vi "CPP-7021Polar.vi"(0 "Plot Array":cluster{dbl[], dbl[]}[](array[cluster])=[{[500.0, 500.0, 953.54, 215.0, 270.0, 320.0, 445.0, 525.0, 600.0, 675.0, 750.0, 825.0, 900.0, 960.0, 1010.0, 1060.0], [4.614524, 4.54365, 5.818368, 0.1374656, 0.6662545, 1.465458, 3.619824, 4.848976, 5.887329, 5.940571, 6.152151, 5.717487, 5.600293, 5.40069, 5.154843, 5.121789]}, {[100.0, 150.0, 215.0, 270.0, 320.0, 445.0, 525.0, 600.0, 675.0, 750.0, 825.0, 900.0, 960.0, 1010.0, 1060.0], [0.002314715, -0.00693192, 0.120417, 0.6880509, 1.519176, 3.513709, 5.065183, 6.116033, 6.096773, 5.938465, 5.593788, 5.5597, 5.387002, 5.304077, 4.887903]}] {"?" format="%.2f"; "?" format="%.2f"}, 1 "Job Directory":path=path "/G4_2_HD/Users/paulhayden/Documents/Projects/Westlakes_resolution") -> (2 "Saved Automatically?":bool, 3 "gnuplotScript":string="set term epslatex\nset output \"Plot.eps\"\nset xlabel '$Distance~(m)$'\nset ylabel '$DF~(s/m^3)\\times10^6$'\nset samples 1000\nset pointsize 1.00\nset title '$B38~Centreline~Glc$' 0, 0\nset size 0.75,0.9\n\n#set key 450, -2.5833\n unset key\nset label 1 '~~~~~~~~~~~Angle~(deg)~=~0' at -100, -2.58\nset label 2 '~~~~~~~~~~~Height~(m)~=~5' at -100, -3.27\n set xrange [0 : 500] \n# set autoscale x \n set yrange [0.10000 : 7]\n# set autoscale y \n\nplot \"B38_Centreline_Glc.dat\" index 0 using 1:2 axes x1y1 title '$File=B38R~DDD.xls$' with points 1 1, \\\n\"B38_Centreline_Glc.dat\" index 1 using 1:2 axes x1y1 title '$File=B38R~DDD~1.xls$' with points 1 3", 4 "Plot data file":path)   [LabVIEW 2015]
uses:
  Results_plotter_Global.vi
panel:
  in  "Tab Control":enum32{"GoodStuff", "OtherStuff"}(tab)
  in  "Margins":dbl=0.6 min=0.1 max=2.0 step=0.1
  out "No of Series":i32=2
  in  "PropertyArray":T1(array[cluster])=[{"Style"="lines", "Color"=16711680, "PointType"=2, "PointSize"=0.6}, {"Style"="points", "Color"=16860, "PointType"=6, "PointSize"=0.6}, {"Style"="points", "Color"=1985280, "PointType"=5, "PointSize"=0.6}, {"Style"="lines", "Color"=0, "PointType"=5, "PointSize"=0.6}] caption="Style                      Colour    PointType       PointSize" {"PointSize" min=0 step=0.1}
  in  "Rows":u8=4 min=1
  in  "Cols":u8=6 min=1
  out "nGraphs":i32
  in  "rmax":dbl=1.1 step=0.1
  in  "rtics":dbl=0.2 step=0.1
  in  "ManualTitles":string[](array[string])=["", "", "", "", "", "", "", "", "", "", "", "", "", "", "", ""]
  in  "Titles":bool=TRUE
  in  "ScaleFactor":dbl
  in  "ScaleAdjust":dbl=0.1 min=0.1 max=2.0 step=0.1
  in  "Legend?":bool
  in  "AngleTics":dbl=30.0 step=0.1
  in  "r Axis?":bool
  in  "Plot Title Pre Block":string
  in  "Plot Title":u16(ring) items=["Title String Only", "Number of Measurements", "TT:used:", "Fence::", "Comments::", "Azimuth::", "ExtraNotes::", "X::", "Y::", "Z_{model}::", "U/Uref::", "U/U(167)::", "(U/Uref)-1::", "V/Uref::", "W/Uref::", "Vmag/Uref::", "Uref::", "U::", "V::", "W::", "Vmag::", "TI:U:%", "TI:V:%", "TI:W:%", "TI:Vmag:%", "Upk/Upk(167)::", "Vmagpk/Uref::", "U_SD::", "V_SD::", "W_SD::", "Vmag_SD::", "Tunnel:X:", "Tunnel:Y:", "5HP:Mode:", "5HP:ReturnType:", "GoodFraction::", "DownstreamEars::", "Ramps::", "Reference:Temperature:Used for Corrections", "Atmos:Pressure:Used for Corrections", "Seconds:since:1st Jan", "Time:Measurement:Commenced", "Multi Run:Start Time:", "Date:of:Measurement", "Run:Messages:", "Current:Data:Filename", "Original:Results:Filename", "Raw:Data:Filename", "P1:mm:", "PostProcessBatch::", "Upk(z=167,Base,AllPts,AllAzs)/Uref::", "U(z=167,Base,AllPts,AllAzs)/Uref::", "Horizontal~Velocity/U_{ref}::", "Z_{fs}:(m):"]
  in  "Plot Title Post Block":string
  out "Array":string[](array[string])
  in  "OpenLogfile?":bool
  in  "Filename Max length":i32=255
  in  "Show Script Editor?":bool
  out "Path":path
  out "Final Title":string="B38 Centreline Glc"
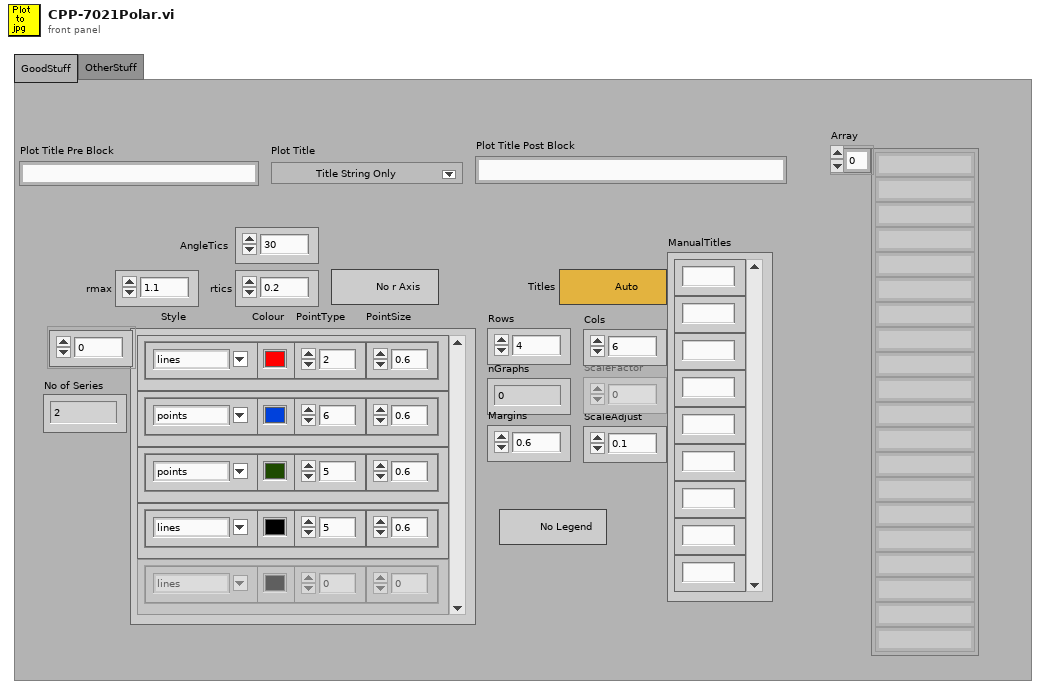
[diagram p1: front panel]
types:
  T1 = cluster{"Style":string, "Color":u32, "PointType":i32, "PointSize":sgl}[]
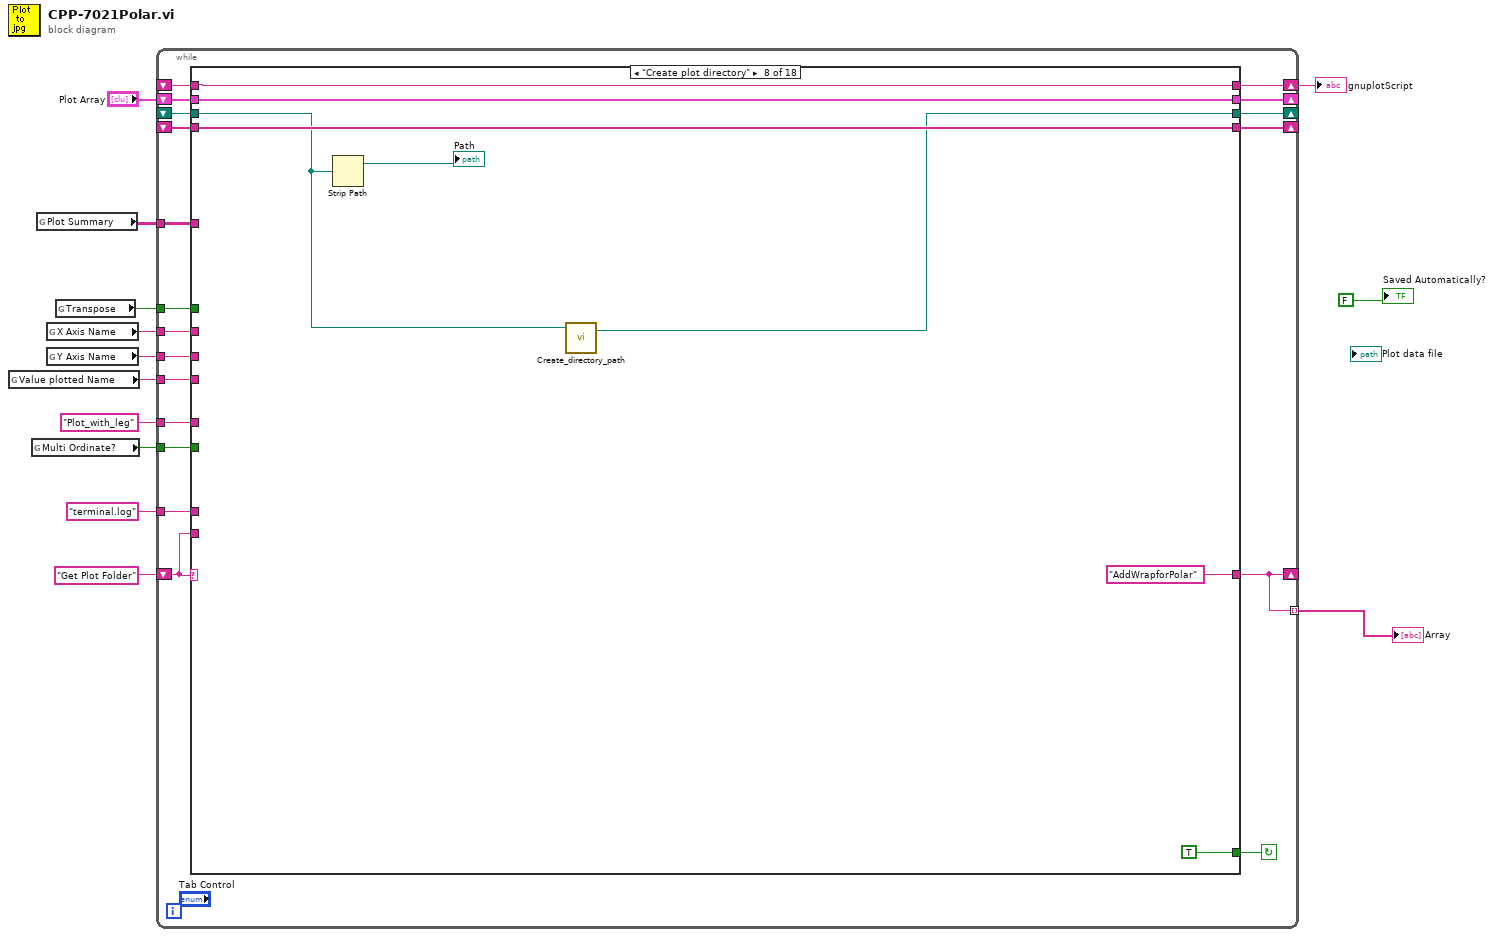
[diagram p0: block diagram]
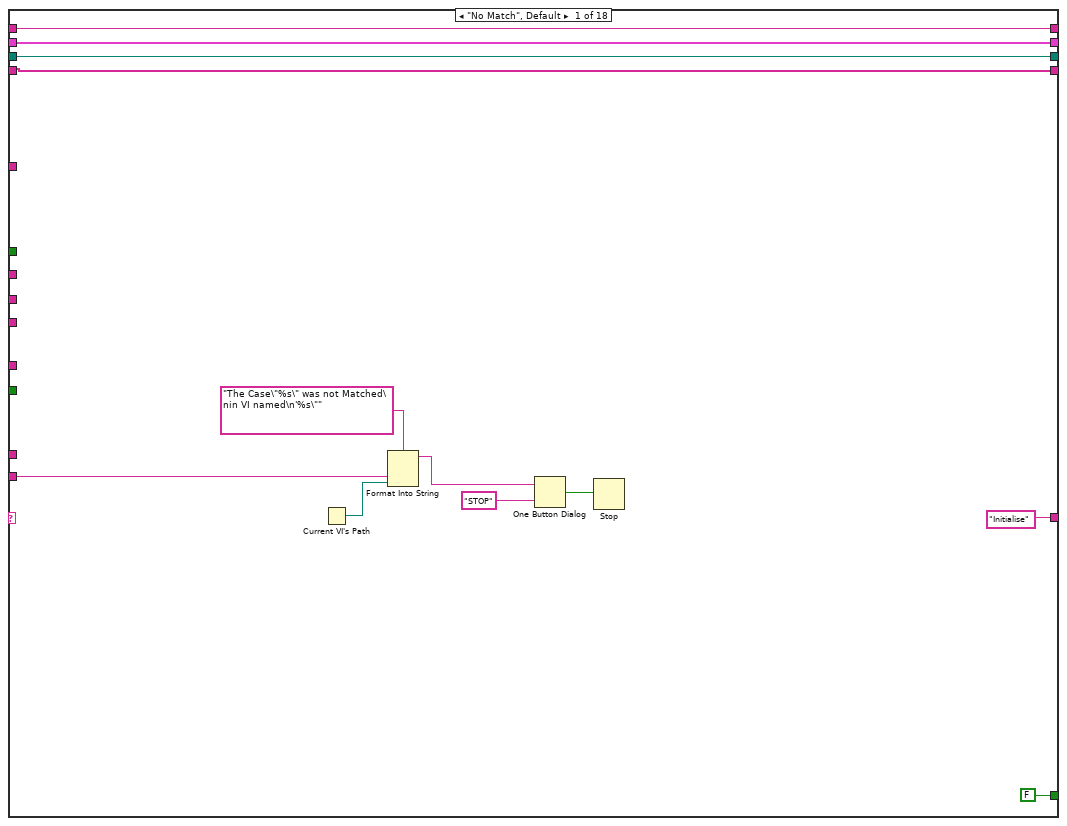
[diagram p2: hidden frame]
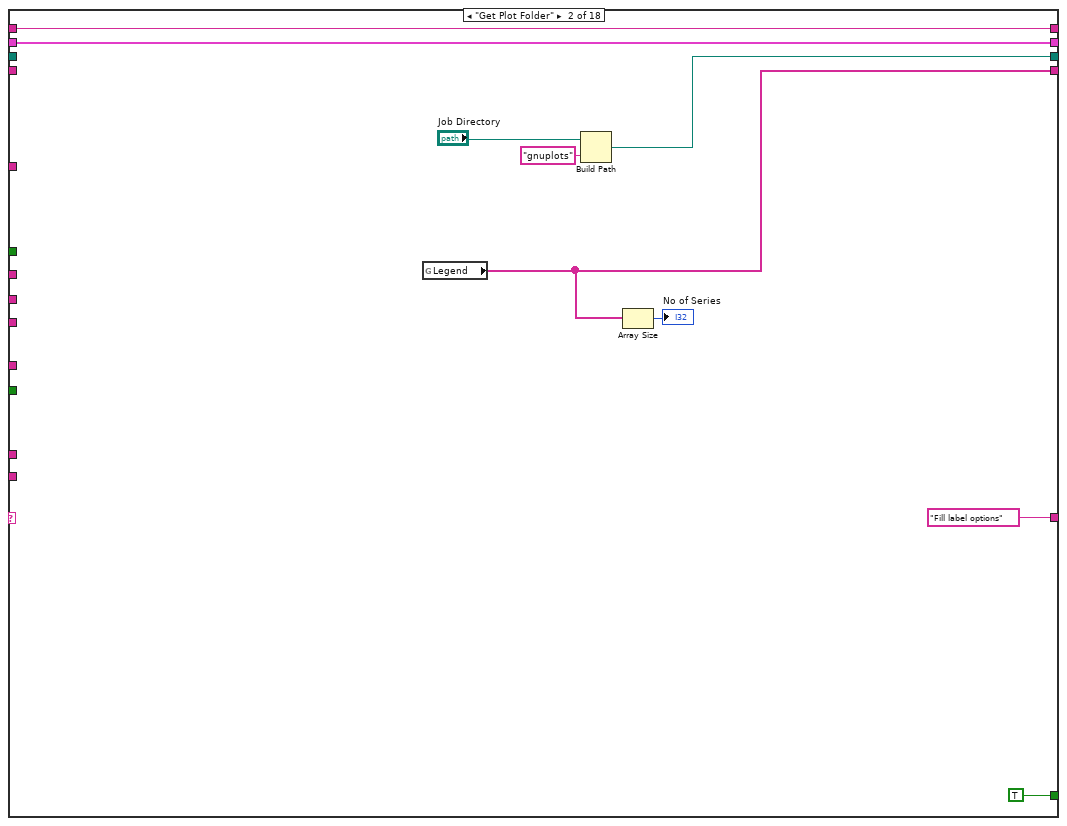
[diagram p3: hidden frame]
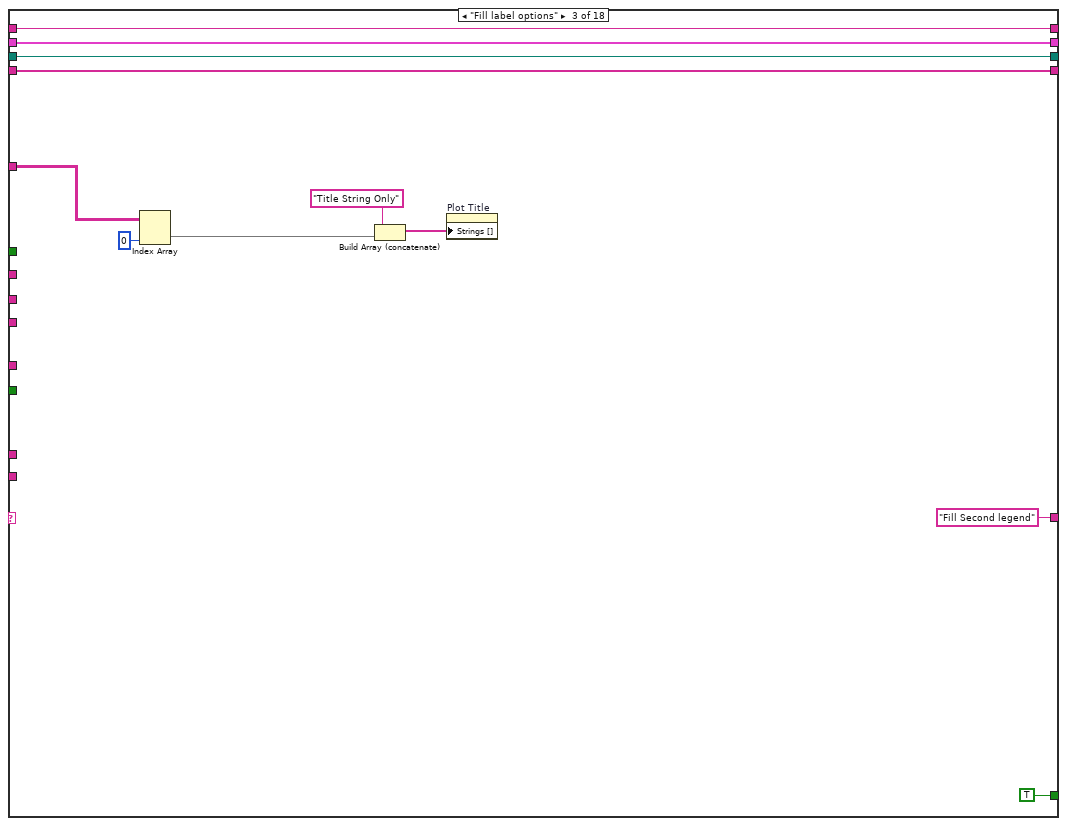
[diagram p4: hidden frame]
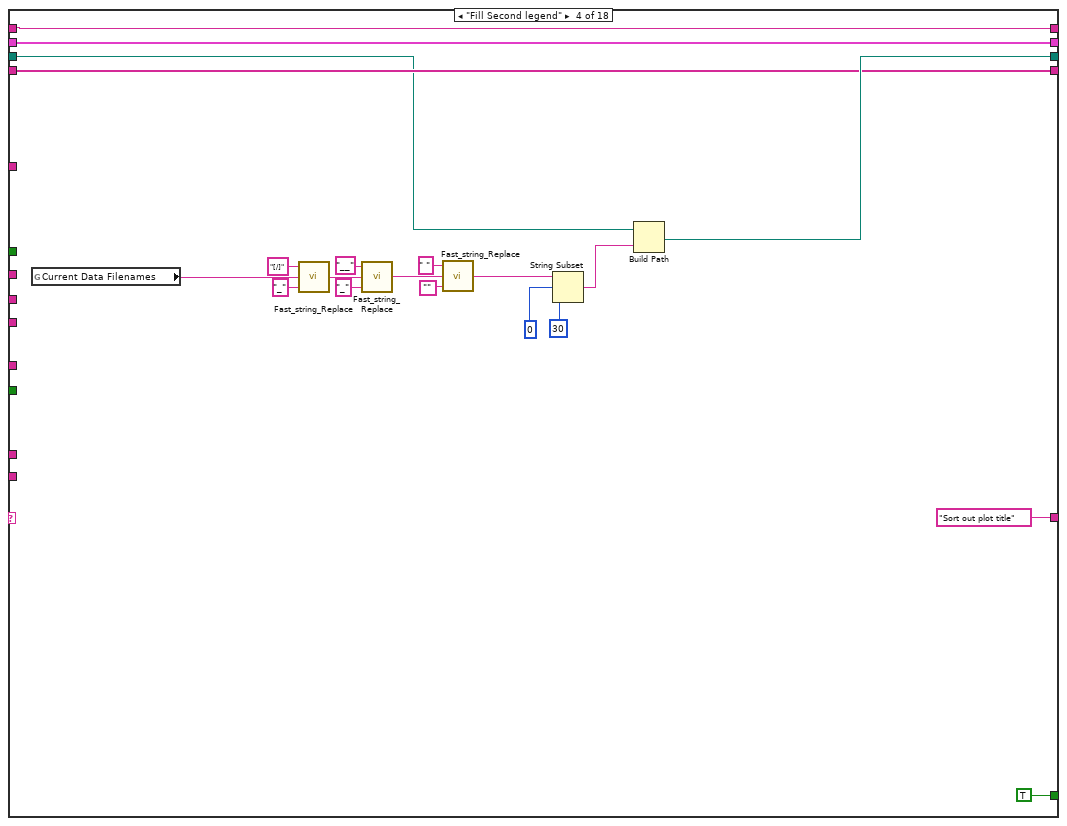
[diagram p5: hidden frame]
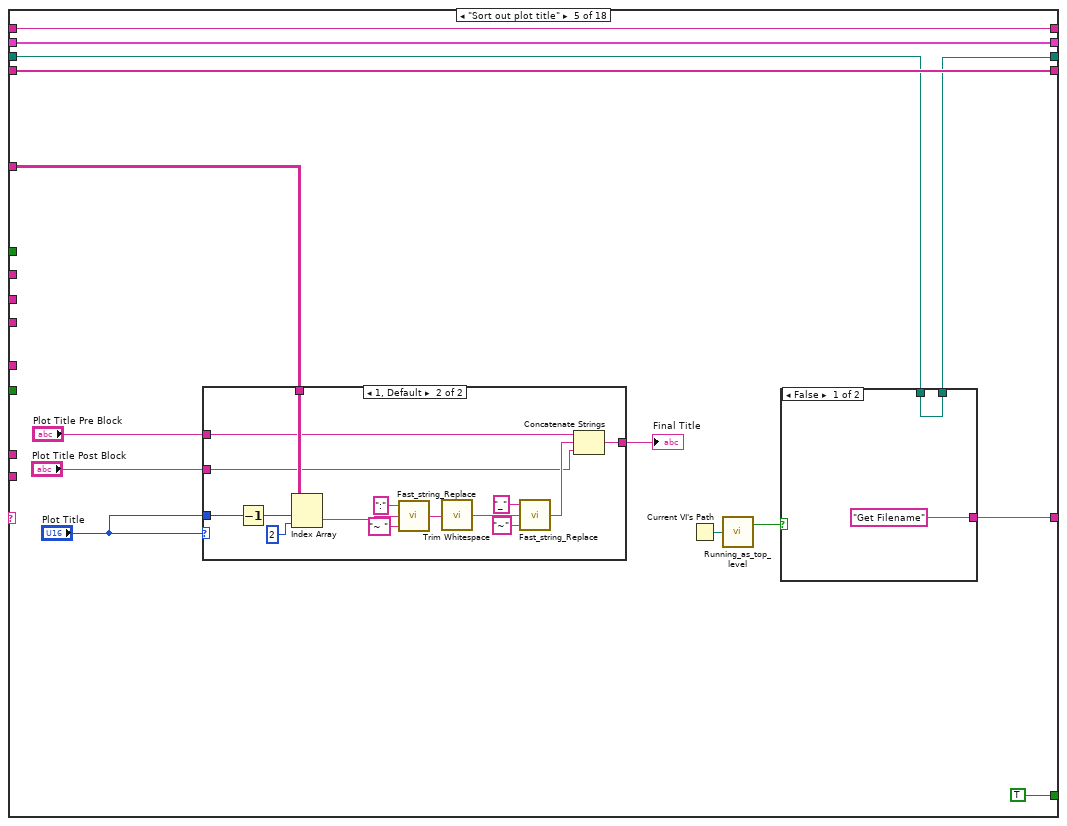
[diagram p6: hidden frame]
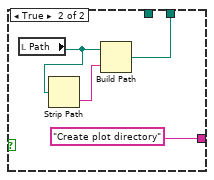
[diagram p7: hidden frame]
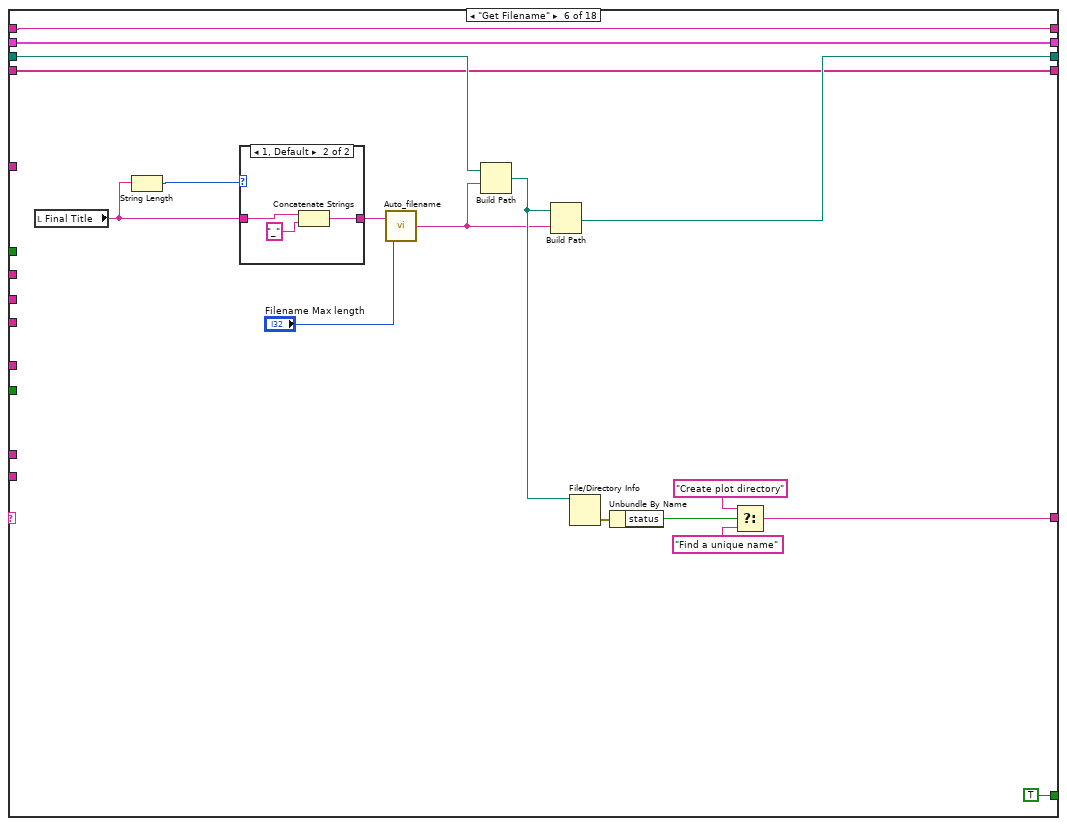
[diagram p9: hidden frame]
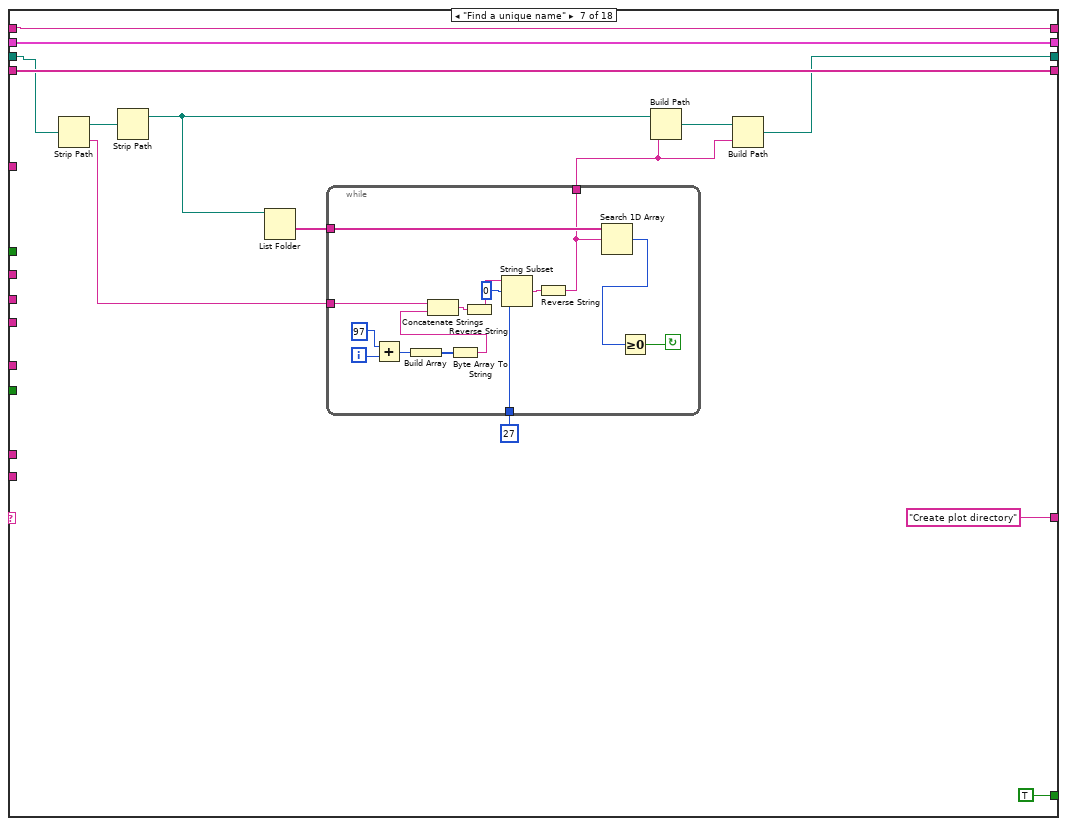
[diagram p11: hidden frame]
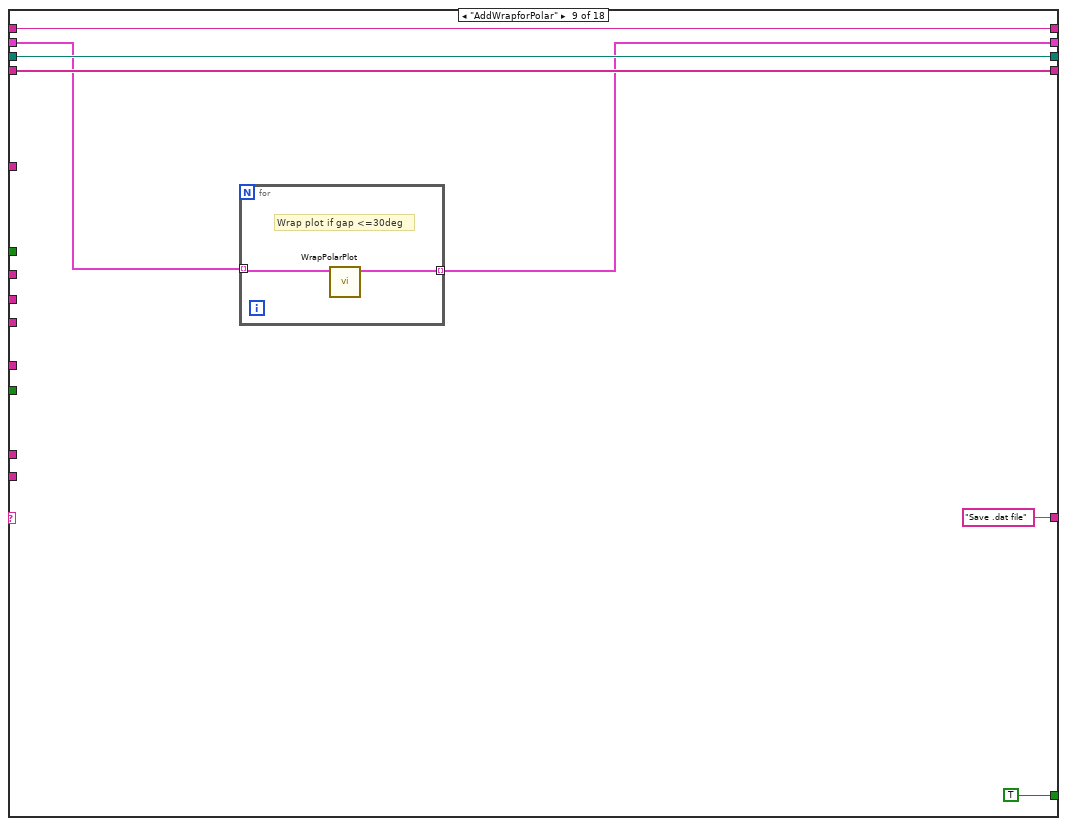
[diagram p12: hidden frame]
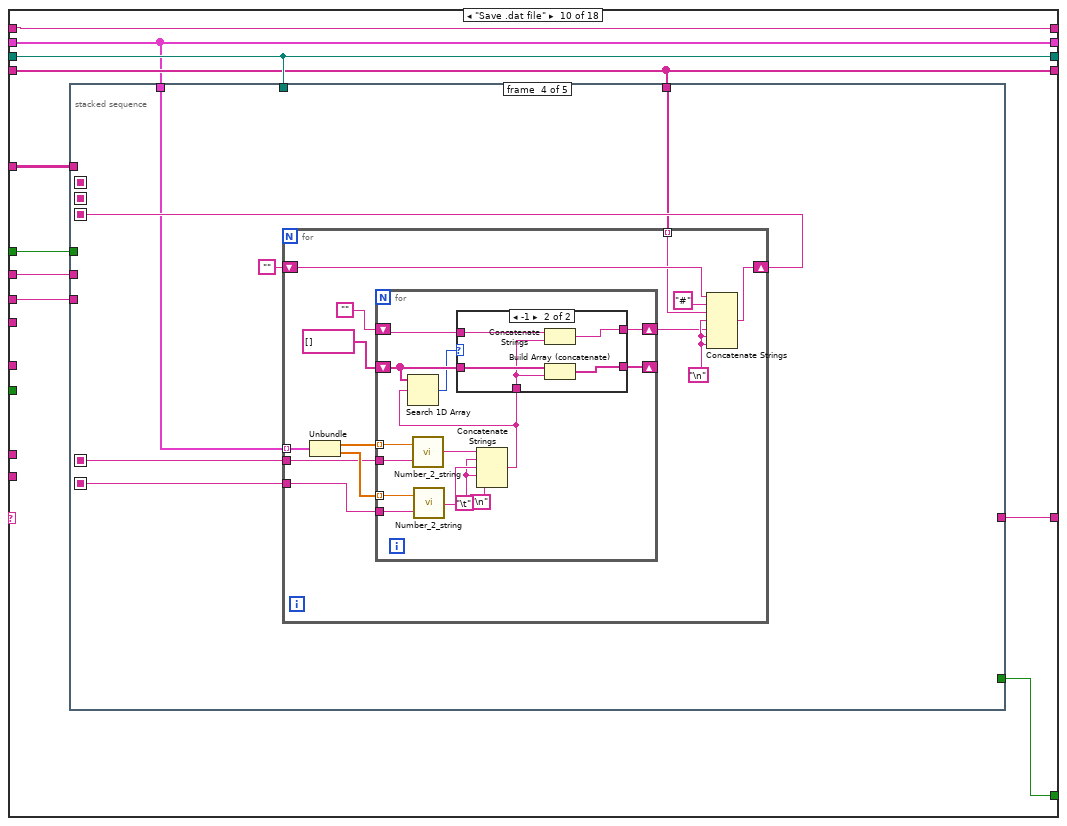
[diagram p13: hidden frame]
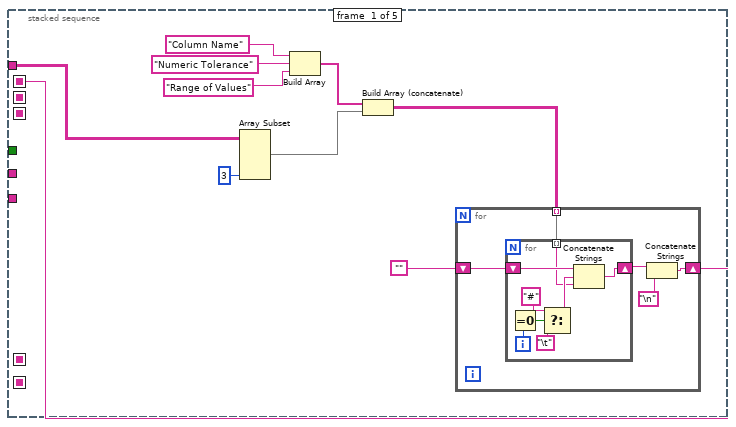
[diagram p14: hidden frame]
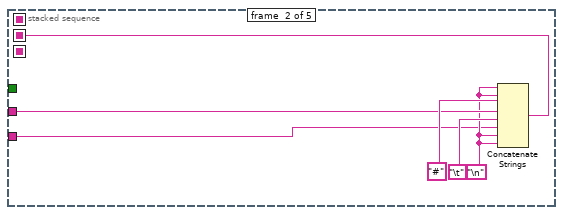
[diagram p15: hidden frame]
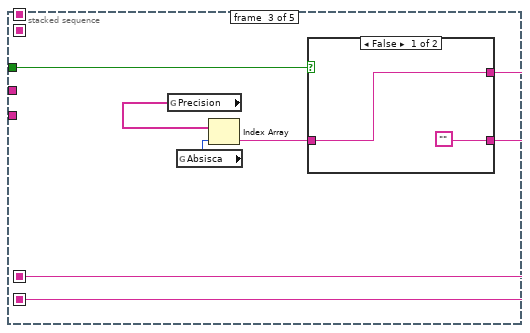
[diagram p16: hidden frame]
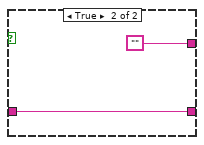
[diagram p17: hidden frame]
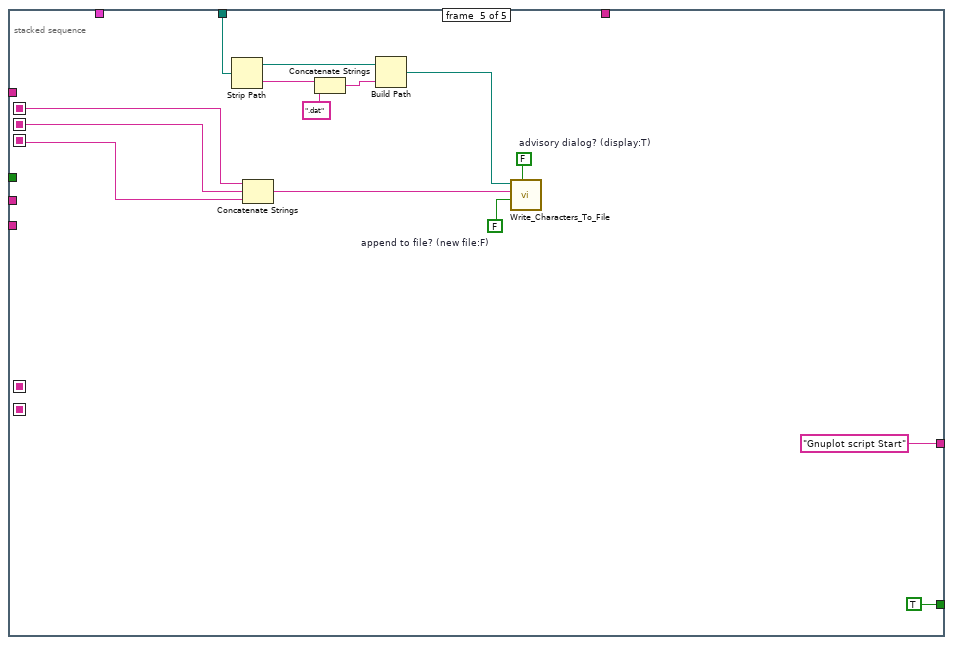
[diagram p19: hidden frame]
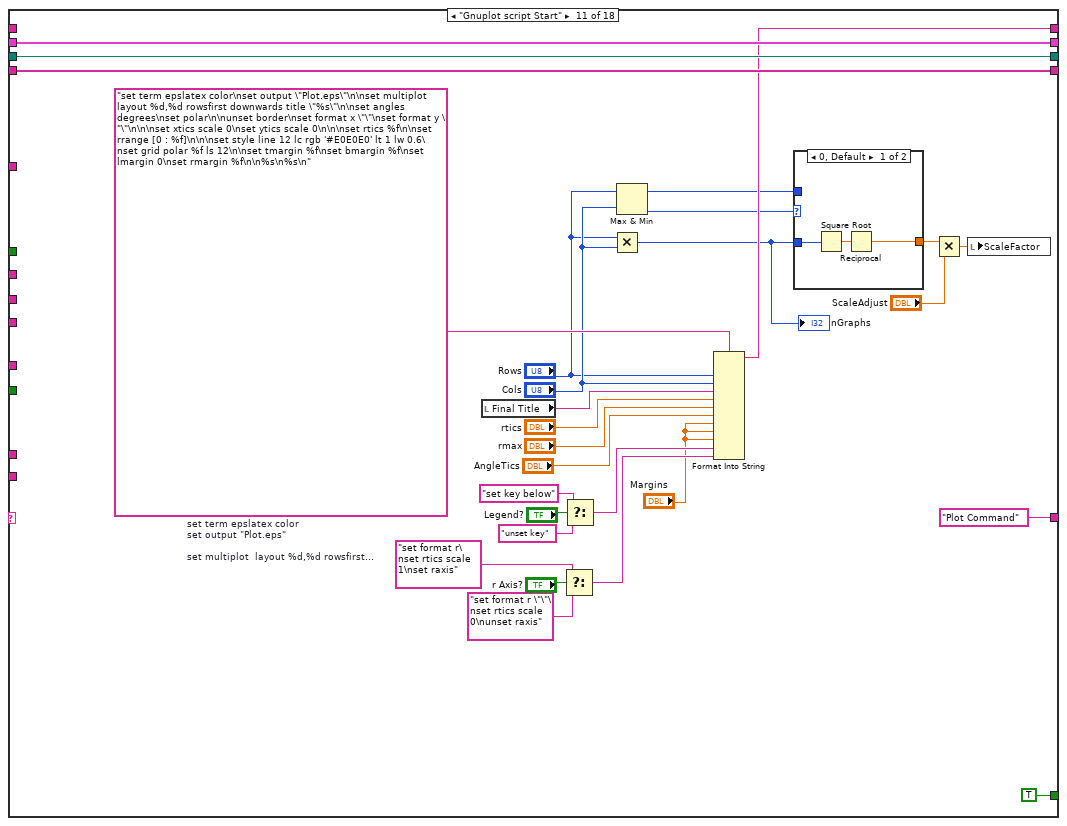
[diagram p20: hidden frame]
diagram:
  n1 = global read "Results_plotter_Global.vi" "Value plotted Name"() -> (w9:string)
  n2 = global read "Results_plotter_Global.vi" "Multi Ordinate?"() -> (w2:bool)
  n3 = global read "Results_plotter_Global.vi" "Plot Summary"() -> (w12:string[][])
  n4 = global read "Results_plotter_Global.vi" "X Axis Name"() -> (w11:string)
  n5 = global read "Results_plotter_Global.vi" "Y Axis Name"() -> (w10:string)
  n6 = global read "Results_plotter_Global.vi" "Transpose"() -> (w3:bool)
  n7 = while {
    shift-left: "Get Plot Folder" -> [w31]
    shift-right: [w14] -> _
    tunnel: w12 -> [w30]
    shift-right: [w29] -> _
    shift-left: _ -> [w28]
    tunnel: w11 -> [w27]
    tunnel: w10 -> [w26]
    tunnel: w9 -> [w25]
    shift-right: [w23] -> _
    shift-left: "Plot Array" -> [w24]
    shift-right: [w21] -> w8
    shift-left: _ -> [w22]
    tunnel: "Plot_with_leg" ("name or relative path") -> [w20]
    shift-right: [w19] -> _
    shift-left: _ -> [w18]
    tunnel: "terminal.log" -> [w17]
    tunnel: w3 -> [w16]
    tunnel: w2 -> [w15]
    tunnel: [w14] -> w1 mode=indexing
    stop <- w32 continue-if-true
    n8 = case shown="\"Create plot directory\"" w31 {
      tunnel: [FALSE TRUE TRUE ("Top Level") TRUE ("Top Level") TRUE ("Top Level") TRUE ("Top Level") TRUE ("Top Level") TRUE TRUE ("Top Level") w195 TRUE ("Top Level") TRUE ("Top Level") TRUE ("Top Level") TRUE ("Top Level") TRUE ("Top Level") FALSE ("Top Level") FALSE ("Top Level") FALSE ("Top Level")] -> w32
      tunnel: ["Initialise" "Fill label options" "Fill Second legend" "Sort out plot title" w86 w135 "Create plot directory" "AddWrapforPolar" "Save .dat file" w194 "Plot Command" "Write gnuplot file" ("t") "Execute shell script" ("t") "Has pdf been generated?" ("t") w429 "End" "End" ("t") "End" ("t")] -> w14
      tunnel: w31 -> [w39 _ _ _ _ _ _ _ _ _ _ _ _ _ _ _ _ _]
      tunnel: w30 -> [_ _ w64 _ w93 _ _ _ _ w193 _ _ _ _ _ _ _ _]
      tunnel: [w36 w50 w58 w84 w88 w136 w142 w175 w184 w196 w317 w341 w411 w419 w433 w438 w448 w454] -> w29
      tunnel: w28 -> [w36 _ w58 w80 w87 w132 w149 w174 w184 w196 w317 w341 w411 w419 w433 w438 w448 w454]
      tunnel: w27 -> [_ _ _ _ _ _ _ _ _ w192 _ _ _ _ _ _ _ _]
      tunnel: w26 -> [_ _ _ _ _ _ _ _ _ w191 _ _ _ _ _ _ _ _]
      tunnel: w25 -> [_ _ _ _ _ _ _ _ _ _ _ _ _ _ _ _ _ _]
      tunnel: w24 -> [w35 w46 w59 w83 w98 w134 w152 w178 w180 w188 w318 w342 w417 w424 w436 w443 w453 w459]
      tunnel: [w35 w46 w59 w83 w98 w134 w152 w178 w179 w188 w318 w342 w417 w424 w436 w443 w453 w459] -> w23
      tunnel: w22 -> [w34 w49 w60 w82 w94 w133 w151 w177 w185 w197 _ w339 w407 w422 w434 w441 w451 w457]
      tunnel: [w34 w49 w60 w82 w94 w133 w151 w177 w185 w197 w312 w338 w407 w422 w434 w441 w451 w457] -> w21
      tunnel: w20 -> [_ _ _ _ _ _ _ _ _ _ _ _ _ _ _ _ _ _]
      tunnel: [w33 w45 w57 w81 w97 w131 w150 w176 w183 w190 w316 w340 w412 w423 w435 w442 w452 w458] -> w19
      tunnel: w18 -> [w33 _ w57 w81 w97 w131 w150 w176 w183 w190 w316 w340 w412 w423 w435 w442 w452 w458]
      tunnel: w17 -> [_ _ _ _ _ _ _ _ _ _ _ _ _ w418 _ _ w446 _]
      tunnel: w16 -> [_ _ _ _ _ _ _ _ _ w189 _ _ _ _ _ _ _ _]
      tunnel: w15 -> [_ _ _ _ _ _ _ _ _ _ _ _ _ _ _ _ _ _]
      frame "No Match", Default {
        n9 = Current VI's Path() -> (path=w38:path)
        n10 = Format Into String(format string="The Case\"%s\" was not Matched\nin VI named\n'%s\"" ("Format String"), w39, w38) -> (resulting string=w42:string)  [unwired: 2 in, 1 out]
        n11 = One Button Dialog(message=w42, button name ("OK")="STOP") -> (true=w40:bool)
        n12 = Stop(stop? (T)=w40) -> ()
      }
      frame "Get Plot Folder" {
        n13 = global read "Results_plotter_Global.vi" "Legend"() -> (w45:string[])
        n14 = Build Path(base path="Job Directory", name or relative path="gnuplots") -> (appended path=w50:path)
        n15 = Array Size(array=w45) -> (size(s)=→"No of Series":i32)
      }
      frame "Fill label options" {
        n16 = Index Array(array=w64, index (col)=0 ("disabled index (col)")) -> (element=w55:string[])  [unwired: 1 in]
        n17 = Build Array (concatenate)("Title String Only", w55) -> (w54:string[])
        n18 = property on="Plot Title" class="Ring (strict)"("Strings []"=w54) -> ()  [unwired: 2 in, 2 out]
      }
      frame "Fill Second legend" {
        n19 = global read "Results_plotter_Global.vi" "Current Data Filenames"() -> (w69:string)
        n20 = call "Fast_string_Replace.vi"("Replace match with:"="_", "Input String"=w69, "regular expression"="[/]") -> ("Output String"=w73:string)  [unwired: 2 out]
        n21 = call "Fast_string_Replace.vi"("Replace match with:"="_", "Input String"=w73, "regular expression"="__") -> ("Output String"=w70:string)  [unwired: 2 out]
        n22 = call "Fast_string_Replace.vi"("Replace match with:"="", "Input String"=w70, "regular expression"=" ") -> ("Output String"=w68:string)  [unwired: 2 out]
        n23 = String Subset(string=w68, offset (0)=0, length (rest)=30 ("length (rest)")) -> (substring=w67:string)
        n24 = Build Path(base path=w80, name or relative path=w67) -> (appended path=w84:path)
      }
      frame "Sort out plot title" {
        n25 = case shown="1, Default" "Plot Title" {
          tunnel: [w105 w110] -> w92
          tunnel: "Plot Title Pre Block" -> [w105 w109]
          tunnel: w93 -> [_ w113]
          tunnel: "Plot Title" -> [_ w112]
          tunnel: "Plot Title Post Block" -> [_ w106]
          frame 0 {
          }
          frame 1, Default {
            n26 = Decrement(x=w112) -> (x-1=w111:u16)
            n27 = Index Array(array=w113, index (row)=w111, index (col)=u16 2 ("y")) -> (element=w116:string)
            n28 = call "Fast_string_Replace.vi"("Replace match with:"="~ ", "Input String"=w116, "regular expression"=":") -> ("Output String"=w115:string)  [unwired: 2 out]
            n29 = call <vilib>:"Trim Whitespace.vi"("string"=w115) -> ("trimmed string"=w114:string)  [unwired: 1 in]
            n30 = call "Fast_string_Replace.vi"("Replace match with:"="~", "Input String"=w114, "regular expression"="_") -> ("Output String"=w108:string)  [unwired: 2 out]
            n31 = Concatenate Strings(w109, w108, w106) -> (w110:string)
          }
        }
        "Final Title" <- w92
        n32 = Current VI's Path() -> (path=w91:path)
        n33 = call "Running_as_top_level.vi"("Vi path name"=w91) -> ("Top Level"=w89:bool)  [unwired: 1 out]
        n34 = case shown="False" w89 {
          tunnel: [w100 w103] -> w88
          tunnel: w87 -> [w100 _]
          tunnel: ["Get Filename" ("t") "Create plot directory"] -> w86
          frame False {
          }
          frame True {
            n35 = local read "Path"() -> (w102:path)
            n36 = Strip Path(path=w102) -> (name=w101:string)  [unwired: 1 out]
            n37 = Build Path(base path=w102, name or relative path=w101) -> (appended path=w103:path)
          }
        }
      }
      frame "Get Filename" {
        n38 = local read "Final Title"() -> (w121:string)
        n39 = String Length(string=w121) -> (length=w123:i32)
        n40 = case shown="1, Default" w123 {
          tunnel: [w138 w139] -> w122
          tunnel: w121 -> [w138 w141]
          frame 0 {
          }
          frame 1, Default {
            n41 = Concatenate Strings(w141, "_") -> (w139:string)
          }
        }
        n42 = call "Auto_filename.vi"("Filename Max length"="Filename Max length", "Prefix"=w122) -> ("Filename"=w125:string)
        n43 = Build Path(base path=w132, name or relative path=w125) -> (appended path=w129:path)
        n44 = Build Path(base path=w129, name or relative path=w125) -> (appended path=w136:path)
        n45 = File/Directory Info(path=w129) -> (error out=w130:errorcluster)  [unwired: 1 in, 6 out]
        n46 = Unbundle By Name(w130) -> ("status"=w128:bool)
        n47 = Select(t="Create plot directory", s=w128, f="Find a unique name") -> (s? t:f=w135:string)
      }
      frame "Find a unique name" {
        n48 = Strip Path(path=w149) -> (stripped path=w148:path, name=w147:string)
        n49 = Strip Path(path=w148) -> (stripped path=w145:path)  [unwired: 1 out]
        n50 = List Folder(path=w145) -> (folder names=w146:string[])  [unwired: 1 in, 5 out]
        n51 = while {
          tunnel: w147 -> [w170]
          tunnel: 27 ("Max Length") -> [w169]
          tunnel: [w158] -> w144
          tunnel: w146 -> [w159]
          i -> [w160]
          stop <- w156 continue-if-true
          n52 = Add(x=97, y=w160) -> (x+y=w167:i32)
          n53 = Build Array(w167) -> (w168:i32[])
          n54 = Byte Array To String(unsigned byte array=w168) -> (string=w165:string)
          n55 = Concatenate Strings(w170, w165) -> (w163:string)
          n56 = Reverse String(1:w163) -> (0:w164:string)
          n57 = String Subset(string=w164, offset (0)=0, length (rest)=w169) -> (substring=w162:string)
          n58 = Reverse String(1:w162) -> (0:w158:string)
          n59 = Search 1D Array(1D array=w159, element=w158) -> (index of element=w157:i32)  [unwired: 1 out]
          n60 = Greater Or Equal To 0?(x=w157) -> (x >= 0?=w156:bool)
        }
        n61 = Build Path(base path=w145, name or relative path=w144) -> (appended path=w143:path)
        n62 = Build Path(base path=w143, name or relative path=w144) -> (appended path=w142:path)
      }
      frame "Create plot directory" {
        n63 = Strip Path(path=w174) -> (stripped path=→"Path":path)  [unwired: 1 out]
        n64 = call "Create_directory_path.vi"("Path name"=w174) -> ("Path name Out"=w175:path)  [unwired: 2 in, 1 out]
      }
      frame "AddWrapforPolar" {
        n65 = for {
          tunnel: w180 -> [w187] mode=indexing
          tunnel: [w186] -> w179 mode=indexing
          # "Wrap plot if gap <=30deg"
          n66 = call "WrapPolarPlot.vi"("thetaRin"=w187) -> ("thetaRout"=w186:cluster{"Angle":dbl[], "Radius":dbl[]})  [unwired: 10 in]
        }
      }
      frame "Save .dat file" {
        n67 = stacked-sequence {
          seq-local: [w198 _ _ _ _] -> [_ _ _ _ w282]
          seq-local: [_ w222 _ _ _] -> [_ _ _ _ w283]
          seq-local: [_ _ _ w241 _] -> [_ _ _ _ w284]
          seq-local: [_ _ w227 _ _] -> [_ _ _ w239 _]
          seq-local: [_ _ w229 _ _] -> [_ _ _ w238 _]
          tunnel: w196 -> [_ _ _ _ w287]
          tunnel: [_ _ _ _ TRUE ("Top Level")] -> w195
          tunnel: [_ _ _ _ "Gnuplot script Start"] -> w194
          tunnel: w193 -> [w203 _ _ _ _]
          tunnel: w192 -> [_ w225 _ _ _]
          tunnel: w191 -> [_ w221 _ _ _]
          tunnel: w188 -> [_ _ _ w237 _]
          tunnel: w190 -> [_ _ _ w240 _]
          tunnel: w189 -> [_ _ w230 _ _]
          frame #0 {
            n68 = Array Subset(array=w203, length (col)=3 ("length")) -> (w201:string[][])  [unwired: 3 in]
            n69 = Build Array("Column Name", "Numeric Tolerance", "Range of Values") -> (w207:string[])
            n70 = Build Array (concatenate)(w207, w201) -> (w199:string[][])
            n71 = for {
              shift-right: [w211] -> w198
              shift-left: "" -> [w208]
              tunnel: w199 -> [w212] mode=indexing
              n72 = for {
                shift-right: [w213] -> w210
                shift-left: w208 -> [w220]
                tunnel: w212 -> [w214] mode=indexing
                i -> [w219]
                n73 = Equal To 0?(x=w219) -> (x = 0?=w218:bool)
                n74 = Select(t="#", s=w218, f="\t") -> (s? t:f=w215:string)
                n75 = Concatenate Strings(w220, w215, w214) -> (w213:string)
              }
              n76 = Concatenate Strings(w210, "\n") -> (w211:string)
            }
          }
          frame #1 {
            w223 = "\n"
            n77 = Concatenate Strings(w223, w223, "#" ("string"), w225, "\t", w221, w223, w223) -> (w222:string)
          }
          frame #2 {
            n78 = global read "Results_plotter_Global.vi" "Precision"() -> (w232:string[])
            n79 = global read "Results_plotter_Global.vi" "Absisca"() -> (w231:i32)
            n80 = Index Array(array=w232, index=w231) -> (element=w228:string)
            n81 = case shown="False" w230 {
              tunnel: ["" w236] -> w229
              tunnel: w228 -> [w233 w236]
              tunnel: [w233 ""] -> w227
              frame False {
              }
              frame True {
              }
            }
          }
          frame #3 {
            n82 = for {
              tunnel: w237 -> [w255] mode=indexing
              shift-right: [w254] -> w241
              shift-left: "" -> [w248]
              tunnel: w240 -> [w246] mode=indexing
              tunnel: w239 -> [w244]
              tunnel: w238 -> [w243]
              w253 = "\n"
              n83 = Unbundle(w255) -> ("Angle"=w249:dbl[], "Radius"=w250:dbl[])
              n84 = for {
                tunnel: w249 -> [w269] mode=indexing
                shift-right: [w264] -> w252
                shift-left: "" -> [w265]
                tunnel: w250 -> [w257] mode=indexing
                shift-right: [w263] -> _
                shift-left: string[] [] -> [w262]
                tunnel: w244 -> [w259]
                tunnel: w243 -> [w258]
                w266 = "\t"
                n85 = call "Number_2_string.vi"("precision"=w259, "number"=w269) -> ("String"=w268:string)
                n86 = call "Number_2_string.vi"("precision"=w258, "number"=w257) -> ("String"=w267:string)
                n87 = Concatenate Strings(w268, w266, w267, w266, "\n") -> (w261:string)
                n88 = Search 1D Array(1D array=w262, element=w261) -> (index of element=w260:i32)  [unwired: 1 in]
                n89 = case shown="-1" w260 {
                  tunnel: w265 -> [w271 w276]
                  tunnel: [w271 w275] -> w264
                  tunnel: w261 -> [_ w272]
                  tunnel: w262 -> [w270 w274]
                  tunnel: [w270 w273] -> w263
                  frame 0, Default {
                  }
                  frame -1 {
                    n90 = Concatenate Strings(w276, w272) -> (w275:string)
                    n91 = Build Array (concatenate)(w274, w272) -> (w273:string[])
                  }
                }
              }
              n92 = Concatenate Strings(w248, "#", w246, w253, w252, w253, w253) -> (w254:string)
            }
          }
          frame #4 {
            w279 = FALSE  # advisory dialog? (display:T)
            w280 = FALSE  # append to file? (new file:F)
            n93 = Strip Path(path=w287) -> (stripped path=w288:path, name=w290:string)
            n94 = Concatenate Strings(w282, w283, w284) -> (w281:string)
            n95 = Concatenate Strings(w290, ".dat" ("string")) -> (w289:string)
            n96 = Build Path(base path=w288, name or relative path=w289) -> (appended path=w278:path)
            n97 = call "Write_Characters_To_File.vi"("file path (dialog if empty)"=w278, "advisory dialog? (display:T)"=w279, "character string"=w281, "append to file? (new file:F)"=w280) -> ()  [unwired: 1 in, 4 out]
          }
        }
      }
      frame "Gnuplot script Start" {
        w313 = "set term epslatex color\nset output \"Plot.eps\"\n\nset multiplot  layout %d,%d rowsfirst downwards title \"%s\"\n\nset angles degrees\nset polar\n\nunset border\nset format x \"\"\nset format y \"\"\n\n\nset xtics scale 0\nset ytics scale 0\n\n\nset rtics %f\n\nset rrange [0 : %f]\n\n\nset style line 12 lc rgb '#E0E0E0' lt 1 lw 0.6\nset grid polar %f ls 12\n\nset tmargin %f\nset bmargin %f\nset lmargin 0\nset rmargin %f\n\n%s\n%s\n"  # set term epslatex color set output "Plot.eps"  set multiplot  layout %d,%d rowsfirst downwards title "%s"  set angles degrees set polar  unset border set format x "" set format y ""   set xtics scale 0 set ytics scale 0   set rtics %f  set rrange [0 : %f]   set style line 12 lc rgb '#E0E0E0' lt 1 lw 0.6 set grid polar %f ls 12  set tmargin %f set bmargin %f set lmargin 0 set rmargin %f  %s %s
        n98 = local read "Final Title"() -> (w311:string)
        n99 = Select(t="set format r\nset rtics scale 1\nset raxis", s="r Axis?", f="set format r \"\"\nset rtics scale 0\nunset raxis") -> (s? t:f=w293:string)
        n100 = Select(t="set key below", s="Legend?", f="unset key") -> (s? t:f=w296:string)
        n101 = Multiply(x="Rows", y="Cols") -> (x*y=w308:u8)
        "nGraphs" <- w308
        n102 = Max & Min(x="Rows", y="Cols") -> (max(x,y)=w303:u8, min(x,y)=w305:u8)
        n103 = Format Into String(format string=w313, "Rows", "Cols", w311, "rtics", "rmax", "AngleTics", "Margins", "Margins", "Margins", w296, w293) -> (resulting string=w312:string)  [unwired: 2 in, 1 out]
        n104 = case shown="0, Default" w305 {
          tunnel: w308 -> [w321 _]
          tunnel: [w319 w322] -> w304
          tunnel: w303 -> [_ w323]
          frame 0, Default {
            n105 = Square Root(x=w321) -> (sqrt(x)=w320:dbl)
            n106 = Reciprocal(x=w320) -> (1/x=w319:dbl)
          }
          frame 1 {
            n107 = Reciprocal(x=w323) -> (1/x=w322:dbl)
          }
        }
        n108 = Multiply(x=w304, y="ScaleAdjust") -> (x*y=w302:dbl)
        n109 = local write "ScaleFactor"(w302) -> ()
      }
      frame "Plot Command" {
        n110 = local read "nGraphs"() -> (w324:i32)
        n111 = Strip Path(path=w341) -> (name=w330:string)  [unwired: 1 out]
        n112 = Array Size(array="PropertyArray") -> (size(s)=w325:i32)
        n113 = for {
          N: w324 -> [_]
          shift-right: [w353] -> w329
          shift-left: "" -> [w361]
          tunnel: w330 -> [w356]
          tunnel: w340 -> [w357]
          tunnel: "PropertyArray" -> [w358]
          tunnel: w325 -> [w351]
          i -> [w349]
          n114 = Multiply(x=w349, y=w351) -> (x*y=w359:i32)
          n115 = for {
            tunnel: w358 -> [w389] mode=indexing
            tunnel: w359 -> [w385]
            tunnel: w357 -> [w386]
            tunnel: w356 -> [w381]
            tunnel: w351 -> [w380]
            shift-right: [w369] -> w354
            shift-left: "" -> [w368]
            tunnel: "\"%s.dat\" index %d using (90-$1):2 axes x1y1 title '%s' w " ("format string") -> [w365]
            i -> [w378]
            n116 = Add(x=w385, y=w378) -> (x+y=w382:i32)
            n117 = Unbundle(w389) -> ("Style"=w364:string, "Color"=w363:u32, "PointType"=w367:i32, "PointSize"=w366:sgl)
            n118 = Index Array(array=w386, index=w382) -> (element=w384:string)
            n119 = case shown="\"Points\"" w364 {
              tunnel: [w396 w400 w406] -> w373
              tunnel: w364 -> [w395 w399 w405]
              tunnel: w363 -> [w394 w398 w404]
              tunnel: w367 -> [w393 _ w403]
              tunnel: w366 -> [w392 _ w402]
              frame "Linespoints", Default {
                n120 = Format Into String(format string=" lc rgb '#%6x' lt -1 pointtype %d pointsize %.1f ", initial string=w395, w394, w393, w392) -> (resulting string=w396:string)  [unwired: 1 in, 1 out]
              }
              frame "Lines" {
                n121 = Format Into String(format string=" lc rgb '#%6x'  lt -1 ", initial string=w399, w398) -> (resulting string=w400:string)  [unwired: 1 in, 1 out]
              }
              frame "Points" {
                n122 = Format Into String(format string=" lc rgb '#%6x' pointtype %d pointsize %.1f ", initial string=w405, w404, w403, w402) -> (resulting string=w406:string)  [unwired: 1 in, 1 out]
              }
            }
            n123 = call "Fast_string_Replace.vi"("Replace match with:"="", "Input String"=w384, "regular expression"="[$]") -> ("Output String"=w383:string)  [unwired: 2 out]
            n124 = Format Into String(format string=w365, initial string="", w381, w382, w383) -> (resulting string=w374:string)  [unwired: 1 in, 1 out]
            n125 = Decrement(x=w380) -> (x-1=w379:i32)
            n126 = Concatenate Strings(w374, w373) -> (w372:string)
            n127 = Concatenate Strings(w374, w373, ",\\" ("string")) -> (w375:string)
            n128 = Equal?(x=w379, y=w378) -> (x = y?=w377:bool)
            n129 = Select(t=w372, s=w377, f=w375) -> (s? t:f=w370:string)
            n130 = Concatenate Strings(w368, w370, "\n") -> (w369:string)
          }
          n131 = Index Array(array="ManualTitles", index=w349) -> (element=w348:string)
          n132 = Increment(x=w349) -> (x+1=w347:i32)
          n133 = Number To Decimal String(number=w347) -> (decimal integer string=w345:string)  [unwired: 1 in]
          n134 = Select(t=w345, s="Titles", f=w348) -> (s? t:f=w344:string)
          n135 = Format Into String(format string="set size square %f\nset title '%s'  offset char 0, char -1\nplot  ", initial string=w361, "ScaleFactor", w344) -> (resulting string=w360:string)  [unwired: 1 in, 1 out]
          n136 = Concatenate Strings(w360, w354) -> (w353:string)
        }
        n137 = Concatenate Strings(w329, "unset multiplot") -> (w327:string)
        n138 = String Length(string=w327) -> (length=w337:i32)
        n139 = Subtract(x=w337, y=4) -> (x-y=w335:i32)
        n140 = String Subset(string=w327, length (rest)=w335) -> (substring=w334:string)  [unwired: 1 out]
        n141 = Concatenate Strings(w339, w334) -> (w338:string)
      }
      frame "Write gnuplot file" {
        w414 = FALSE  # append to file? (new file:F)
        w415 = FALSE  # advisory dialog? (display:T)
        n142 = Strip Path(path=w411) -> (stripped path=w408:path)  [unwired: 1 out]
        n143 = Build Path(base path=w408, name or relative path="gnuplot_script.txt") -> (appended path=w416:path)
        n144 = call "Write_Characters_To_File.vi"("file path (dialog if empty)"=w416, "advisory dialog? (display:T)"=w415, "character string"=w407, "append to file? (new file:F)"=w414) -> ()  [unwired: 1 in, 4 out]
      }
      frame "Execute shell script" {
        n145 = call "Run_Gnuplot_Script.vi"("logfileName"=w418, "workingDirectory"=w419) -> ()  [unwired: 1 in]
      }
      frame "Has pdf been generated?" {
        n146 = Select(t="Open Standard output file" ("f"), s="OpenLogfile?", f="End") -> (s? t:f=w427:string)
        n147 = Select(t="Show Re-Run Gnuplot?", s="Show Script Editor?", f=w427) -> (s? t:f=w429:string)
      }
      frame "Show Re-Run Gnuplot?" {
        n148 = Strip Path(path=w438) -> (stripped path=w437:path)  [unwired: 1 out]
        n149 = call "Re_run_Gnuplot.vi"("Plot folder (dialog if empty)"=w437) -> ()  [unwired: 1 in, 3 out]
      }
      frame "Open Standard output file" {
        n150 = Strip Path(path=w448) -> (stripped path=w445:path)  [unwired: 1 out]
        n151 = Format Into String(format string="open \"%s\"", w446) -> (resulting string=w444:string)  [unwired: 2 in, 1 out]
        n152 = call <vilib>:"System Exec.vi"("working directory"=w445, "command line"=w444) -> ()  [unwired: 4 in, 6 out]
      }
      frame "End" {
      }
    }
  }
  "gnuplotScript" <- w8
  "Array" <- w1
  "Saved Automatically?" <- FALSE
